vi "RichToFlatni_measurementlink_pinmap_v1_RelayGroupDefinition.vi"(5 "OutputClusterType":T1, 11 "InputCluster":T2) -> (3 "OutputCluster":T1)   [LabVIEW 2020, in "Measurement Plugin Pin Map Client.lvlib"]
uses:
  Measurement Plugin Pin Map Client.lvlib
  ni_measurementlink_pinmap_v1_RelayGroupDefinition.ctl
  ni_measurementlink_pinmap_v1_RelayGroupDefinition_Flat.ctl
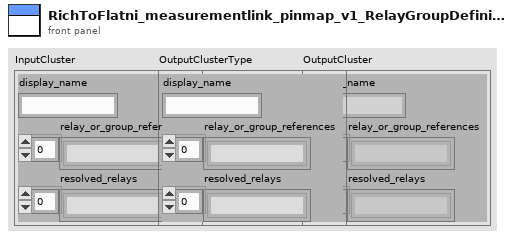
[diagram p1: front panel]
types:
  T1 = typedef "Measurement Plugin Pin Map Client.lvlib/ni_measurementlink_pinmap_v1_RelayGroupDefinition_Flat.ctl" = cluster{"display_name":string, "relay_or_group_references":string[], "resolved_relays":string[]}
  T2 = typedef "Measurement Plugin Pin Map Client.lvlib/ni_measurementlink_pinmap_v1_RelayGroupDefinition.ctl" = cluster{"display_name":string, "relay_or_group_references":string[], "resolved_relays":string[]}
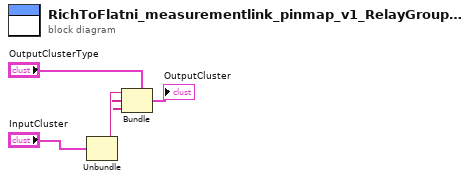
[diagram p0: block diagram]
diagram:
  n1 = Unbundle "Unbundle"("InputCluster") -> ("display_name"=w3:string, "relay_or_group_references"=w2:string[], "resolved_relays"=w1:string[])
  n2 = Bundle "Bundle"(cluster="OutputClusterType", "display_name"=w3, "relay_or_group_references"=w2, "resolved_relays"=w1) -> (→"OutputCluster":T1)
